vi "Set Multiple Attributes to Variant.vi"(8 "error in":errorcluster, 9 "Values":variant[](array[variant]), 10 "Keys":string[](array[string]), 11 "Variant in":variant) -> (0 "error out":errorcluster, 3 "Variant out":variant)   [LabVIEW 2020, in "hse-misc.lvlib"]
doc: "Set multiple attributes (key-values-pairs) to a variant.\n\n____\nHAMPEL SOFTWARE ENGINEERING v3.8.0 (2023-12-18 14:41)"
uses:
  hse-misc.lvlib
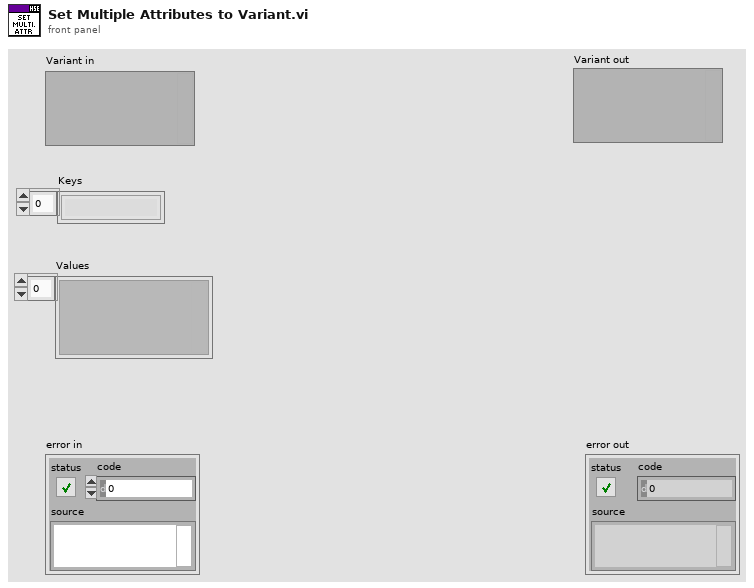
[diagram p1: front panel]
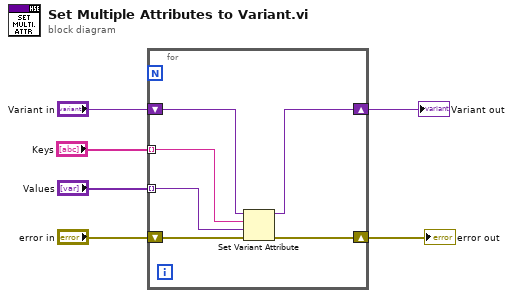
[diagram p0: block diagram]
diagram:
  n1 = for {
    shift-right: [w10] -> w3
    shift-left: "Variant in" -> [w11]
    shift-right: [w9] -> w4
    shift-left: "error in" -> [w12]
    tunnel: "Keys" -> [w8] mode=indexing
    tunnel: "Values" -> [w7] mode=indexing
    n2 = Set Variant Attribute(Variant=w11, name=w8, value=w7, error in=w12) -> (Variant out=w10:variant, error out=w9:errorcluster)  [unwired: 1 out]
  }
  "error out" <- w4
  "Variant out" <- w3
